vi "Write Encoded UTF-8 Path.vi"(10 "Encoded UTF-8 Path":T1) -> (2 "UTF-8 Path":refnum<class "UTF-8 Path.lvclass">)   [LabVIEW 2020, in "G-Unicode.lvlib" / "UTF-8 Path.lvclass"]
doc: "Set the UTF-8 path with an already encoded LabVIEW path.\n\nThe LabVIEW path is assumed to be UTF-8 encoded. Use <b>New UTF-8 Path.vi</b> for converting a LabVIEW path to a UTF-8 path."
uses:
  UTF-8 Path.lvclass
  Encoded UTF-8 Path.ctl
  UTF-8 Path.lvclass/UTF-8 Path.ctl
  G-Unicode.lvlib
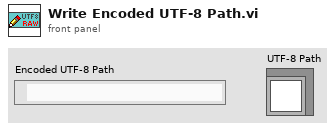
[diagram p1: front panel]
types:
  T1 = typedef "G-Unicode.lvlib/Encoded UTF-8 Path.ctl" = path
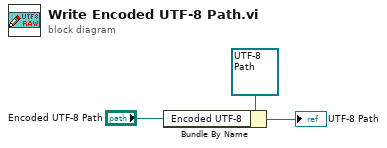
[diagram p0: block diagram]
diagram:
  n1 = Bundle By Name(cluster=refnum<class "UTF-8 Path.lvclass"> refnum ("G-Unicode.lvlib:UTF-8.lvclass"), "Encoded UTF-8"="Encoded UTF-8 Path") -> (→"UTF-8 Path":refnum<class "UTF-8 Path.lvclass">)
